vi "Update All.vi"(0 "reference in":refnum<class "DI.lvclass">, 5 "error in (no error)":errorcluster) -> (14 "reference out":refnum<class "DI.lvclass">, 19 "error out":errorcluster)   [LabVIEW 2017, in "DI.lvclass"]
uses:
  DI.lvclass
  <vilib>/DAQmx/read.llb/DAQmx Read (Digital 1D Bool NChan 1Samp 1Line).vi
  <vilib>/DAQmx/miscellaneous.llb/DAQmx Fill In Error Info.vi
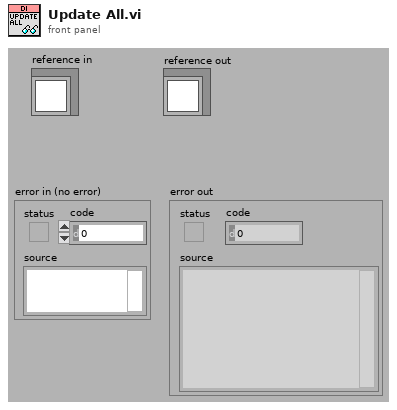
[diagram p1: front panel]
types:
  T1 = typedef "DI.lvclass/ObjectAttributes.ctl" = cluster{"DI Task":refnum<k21>, "DI Status":bool[], "DI Module Names (NI-Max Name)":string[], "Number of Channels Per DI Module":i32[], "Number of DI Modules":u32, "Number of Total DI Channels":u32, "DI On/Off Status":bool, "DO VI Reference":refnum<vi>}
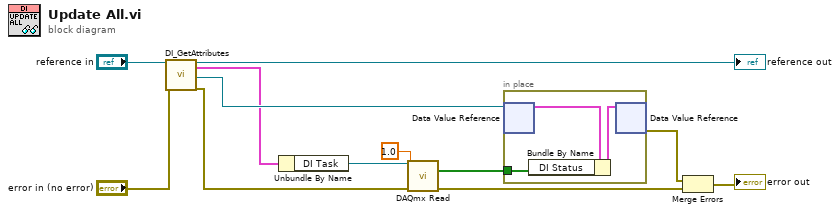
[diagram p0: block diagram]
diagram:
  n1 = call "DI_GetAttributes.vi"("reference in"="reference in", "error in (no error)"="error in (no error)") -> ("reference out"=→"reference out":refnum<class "DI.lvclass">, "Data"=w5:T1, "DataRef"=w8:refnum<data-value>, "error out"=w2:errorcluster)  [unwired: 14 in]
  n2 = Unbundle By Name(w5) -> ("DI Task"=w3:refnum<k21>)
  n3 = call-poly <vilib>:"DAQmx Read.vi"("task/channels in"=w3, "timeout"=1.0, "error in"=w2) -> ("data"=w6:bool[], "error out"=w4:errorcluster)  [unwired: 10 in, 1 out]
  n4 = in-place {
    in-place-border: w6 -> [w13]
    n5 = in-place-dvr #1(w8) -> (w14:T1)  [unwired: 1 out]
    n6 = Bundle By Name(cluster=w14, "DI Status"=w13) -> (w15:T1)
    n7 = in-place-dvr #1(w15) -> (w7:errorcluster)  [unwired: 1 out]
  }
  n8 = Merge Errors(w7, w4) -> (→"error out":errorcluster)
